vi "MNIST_weight print_OLED_sub.vi"(1 "최소값":dbl=-255.0, 2 "최대값":dbl=255.0, 3 "배열":dbl[][](array[numeric])=[[139.0, 142.0, 145.0, 142.0, 138.0, 139.0, 139.0, 139.0, 139.0, 142.0, 144.0, 141.0, 136.0, 140.0, 145.0, 145.0, 145.0, 145.0, 145.0, 144.0, 141.0, 139.0, 142.0, 144.0, 146.0, 147.0, 142.0, 143.0], [140.0, 138.0, 145.0, 143.0, 144.0, 146.0, 141.0, 136.0, 133.0, 128.0, 125.0, 113.0, 121.0, 115.0, 124.0, 119.0, 122.0, 120.0, 128.0, 126.0, 119.0, 119.0, 122.0, 119.0, 142.0, 138.0, 146.0, 141.0], [142.0, 138.0, 138.0, 124.0, 126.0, 139.0, 135.0, 126.0, 125.0, 125.0, 108.0, 106.0, 104.0, 105.0, 107.0, 105.0, 105.0, 95.0, 111.0, 108.0, 114.0, 117.0, 117.0, 114.0, 144.0, 145.0, 139.0, 141.0], [141.0, 139.0, 144.0, 120.0, 125.0, 121.0, 123.0, 114.0, 118.0, 113.0, 91.0, 75.0, 54.0, 54.0, 35.0, 37.0, 51.0, 92.0, 132.0, 131.0, 108.0, 104.0, 127.0, 131.0, 133.0, 141.0, 143.0, 142.0], [138.0, 138.0, 143.0, 128.0, 142.0, 119.0, 109.0, 82.0, 79.0, 51.0, 46.0, 87.0, 87.0, 91.0, 98.0, 84.0, 77.0, 80.0, 88.0, 11.0, 9.0, 24.0, 68.0, 80.0, 105.0, 134.0, 135.0, 138.0], [138.0, 143.0, 144.0, 124.0, 121.0, 92.0, 54.0, 107.0, 125.0, 115.0, 127.0, 153.0, 148.0, 149.0, 131.0, 138.0, 113.0, 121.0, 123.0, 128.0, 130.0, 117.0, 104.0, 12.0, 36.0, 95.0, 118.0, 136.0], [147.0, 130.0, 114.0, 116.0, 93.0, 73.0, 115.0, 125.0, 129.0, 145.0, 145.0, 155.0, 156.0, 162.0, 162.0, 154.0, 161.0, 165.0, 163.0, 147.0, 149.0, 139.0, 124.0, 100.0, 95.0, 120.0, 99.0, 121.0], [143.0, 115.0, 108.0, 95.0, 81.0, 95.0, 125.0, 120.0, 141.0, 146.0, 145.0, 150.0, 159.0, 170.0, 166.0, 174.0, 170.0, 155.0, 150.0, 151.0, 147.0, 146.0, 137.0, 130.0, 100.0, 96.0, 88.0, 113.0], [129.0, 96.0, 89.0, 92.0, 110.0, 127.0, 137.0, 125.0, 148.0, 137.0, 140.0, 134.0, 133.0, 151.0, 160.0, 157.0, 148.0, 148.0, 145.0, 143.0, 137.0, 151.0, 133.0, 118.0, 113.0, 97.0, 88.0, 127.0], [122.0, 109.0, 83.0, 116.0, 119.0, 139.0, 151.0, 144.0, 146.0, 141.0, 150.0, 142.0, 145.0, 146.0, 152.0, 156.0, 142.0, 143.0, 146.0, 140.0, 141.0, 129.0, 133.0, 117.0, 119.0, 96.0, 88.0, 114.0], [126.0, 110.0, 84.0, 120.0, 126.0, 145.0, 152.0, 145.0, 147.0, 145.0, 146.0, 148.0, 149.0, 134.0, 137.0, 134.0, 141.0, 144.0, 146.0, 139.0, 142.0, 138.0, 135.0, 124.0, 101.0, 121.0, 90.0, 116.0], [123.0, 107.0, 95.0, 117.0, 133.0, 153.0, 150.0, 148.0, 162.0, 153.0, 157.0, 162.0, 142.0, 136.0, 142.0, 153.0, 157.0, 159.0, 158.0, 153.0, 163.0, 157.0, 149.0, 127.0, 106.0, 106.0, 107.0, 125.0], [129.0, 97.0, 102.0, 122.0, 159.0, 155.0, 158.0, 154.0, 153.0, 157.0, 158.0, 151.0, 127.0, 144.0, 149.0, 159.0, 159.0, 167.0, 159.0, 161.0, 160.0, 158.0, 152.0, 164.0, 85.0, 43.0, 92.0, 124.0], [132.0, 112.0, 103.0, 130.0, 176.0, 158.0, 154.0, 155.0, 155.0, 149.0, 152.0, 139.0, 127.0, 146.0, 156.0, 158.0, 169.0, 160.0, 161.0, 163.0, 158.0, 161.0, 150.0, 125.0, 53.0, 76.0, 111.0, 138.0], [124.0, 122.0, 97.0, 148.0, 159.0, 139.0, 152.0, 150.0, 143.0, 145.0, 145.0, 139.0, 135.0, 148.0, 145.0, 160.0, 163.0, 161.0, 152.0, 152.0, 158.0, 151.0, 142.0, 102.0, 32.0, 101.0, 124.0, 140.0], [125.0, 146.0, 91.0, 140.0, 142.0, 145.0, 143.0, 142.0, 150.0, 137.0, 147.0, 149.0, 138.0, 136.0, 137.0, 151.0, 158.0, 156.0, 149.0, 148.0, 146.0, 142.0, 141.0, 107.0, 48.0, 96.0, 136.0, 125.0], [126.0, 132.0, 109.0, 132.0, 142.0, 144.0, 134.0, 145.0, 147.0, 132.0, 148.0, 149.0, 139.0, 135.0, 137.0, 148.0, 159.0, 159.0, 151.0, 134.0, 134.0, 126.0, 140.0, 115.0, 48.0, 72.0, 115.0, 113.0], [140.0, 124.0, 113.0, 124.0, 112.0, 122.0, 131.0, 145.0, 145.0, 143.0, 147.0, 143.0, 143.0, 137.0, 142.0, 154.0, 146.0, 146.0, 142.0, 140.0, 134.0, 131.0, 126.0, 109.0, 58.0, 105.0, 119.0, 115.0], [150.0, 127.0, 113.0, 108.0, 95.0, 110.0, 135.0, 140.0, 138.0, 133.0, 156.0, 149.0, 126.0, 128.0, 152.0, 150.0, 138.0, 143.0, 133.0, 135.0, 140.0, 125.0, 127.0, 99.0, 54.0, 104.0, 104.0, 123.0], [144.0, 119.0, 81.0, 113.0, 105.0, 115.0, 132.0, 143.0, 132.0, 117.0, 130.0, 123.0, 128.0, 134.0, 132.0, 132.0, 135.0, 133.0, 129.0, 139.0, 139.0, 126.0, 121.0, 113.0, 93.0, 121.0, 121.0, 127.0], [138.0, 124.0, 108.0, 119.0, 122.0, 129.0, 121.0, 116.0, 129.0, 110.0, 101.0, 108.0, 114.0, 129.0, 128.0, 126.0, 134.0, 134.0, 125.0, 134.0, 127.0, 113.0, 126.0, 125.0, 149.0, 163.0, 115.0, 142.0], [142.0, 124.0, 106.0, 97.0, 137.0, 138.0, 126.0, 127.0, 133.0, 137.0, 133.0, 124.0, 124.0, 127.0, 131.0, 132.0, 132.0, 126.0, 125.0, 125.0, 131.0, 135.0, 124.0, 126.0, 154.0, 141.0, 116.0, 141.0], [141.0, 138.0, 91.0, 127.0, 143.0, 126.0, 127.0, 127.0, 147.0, 146.0, 150.0, 146.0, 146.0, 138.0, 144.0, 129.0, 137.0, 128.0, 125.0, 118.0, 136.0, 134.0, 143.0, 151.0, 149.0, 141.0, 105.0, 143.0], [144.0, 146.0, 107.0, 132.0, 112.0, 128.0, 123.0, 133.0, 145.0, 135.0, 144.0, 139.0, 140.0, 138.0, 142.0, 137.0, 133.0, 138.0, 133.0, 139.0, 144.0, 146.0, 164.0, 161.0, 152.0, 122.0, 115.0, 138.0], [147.0, 142.0, 120.0, 97.0, 138.0, 153.0, 143.0, 152.0, 143.0, 127.0, 140.0, 130.0, 134.0, 124.0, 127.0, 139.0, 138.0, 146.0, 141.0, 140.0, 154.0, 148.0, 162.0, 172.0, 129.0, 113.0, 122.0, 142.0], [144.0, 146.0, 161.0, 97.0, 143.0, 175.0, 160.0, 153.0, 161.0, 148.0, 151.0, 143.0, 144.0, 150.0, 152.0, 145.0, 152.0, 150.0, 160.0, 156.0, 180.0, 174.0, 142.0, 146.0, 127.0, 124.0, 124.0, 141.0], [140.0, 146.0, 142.0, 158.0, 183.0, 178.0, 184.0, 180.0, 175.0, 178.0, 169.0, 168.0, 176.0, 172.0, 183.0, 161.0, 165.0, 168.0, 174.0, 159.0, 170.0, 154.0, 145.0, 151.0, 152.0, 132.0, 147.0, 138.0], [141.0, 145.0, 138.0, 145.0, 116.0, 115.0, 145.0, 150.0, 153.0, 150.0, 143.0, 142.0, 144.0, 96.0, 150.0, 141.0, 132.0, 110.0, 139.0, 123.0, 146.0, 133.0, 123.0, 118.0, 147.0, 138.0, 147.0, 140.0], [138.0, 0.0, 0.0, 0.0, 0.0, 0.0, 0.0, 0.0, 0.0, 0.0, 0.0, 0.0, 0.0, 0.0, 0.0, 0.0, 0.0, 0.0, 0.0, 0.0, 0.0, 0.0, 0.0, 0.0, 0.0, 0.0, 0.0, 0.0]]) -> (0 "MNIST_Input":dbl[][](graph)=[[139.0, 142.0, 145.0, 142.0, 138.0, 139.0, 139.0, 139.0, 139.0, 142.0, 144.0, 141.0, 136.0, 140.0, 145.0, 145.0, 145.0, 145.0, 145.0, 144.0, 141.0, 139.0, 142.0, 144.0, 146.0, 147.0, 142.0, 143.0], [140.0, 138.0, 145.0, 143.0, 144.0, 146.0, 141.0, 136.0, 133.0, 128.0, 125.0, 113.0, 121.0, 115.0, 124.0, 119.0, 122.0, 120.0, 128.0, 126.0, 119.0, 119.0, 122.0, 119.0, 142.0, 138.0, 146.0, 141.0], [142.0, 138.0, 138.0, 124.0, 126.0, 139.0, 135.0, 126.0, 125.0, 125.0, 108.0, 106.0, 104.0, 105.0, 107.0, 105.0, 105.0, 95.0, 111.0, 108.0, 114.0, 117.0, 117.0, 114.0, 144.0, 145.0, 139.0, 141.0], [141.0, 139.0, 144.0, 120.0, 125.0, 121.0, 123.0, 114.0, 118.0, 113.0, 91.0, 75.0, 54.0, 54.0, 35.0, 37.0, 51.0, 92.0, 132.0, 131.0, 108.0, 104.0, 127.0, 131.0, 133.0, 141.0, 143.0, 142.0], [138.0, 138.0, 143.0, 128.0, 142.0, 119.0, 109.0, 82.0, 79.0, 51.0, 46.0, 87.0, 87.0, 91.0, 98.0, 84.0, 77.0, 80.0, 88.0, 11.0, 9.0, 24.0, 68.0, 80.0, 105.0, 134.0, 135.0, 138.0], [138.0, 143.0, 144.0, 124.0, 121.0, 92.0, 54.0, 107.0, 125.0, 115.0, 127.0, 153.0, 148.0, 149.0, 131.0, 138.0, 113.0, 121.0, 123.0, 128.0, 130.0, 117.0, 104.0, 12.0, 36.0, 95.0, 118.0, 136.0], [147.0, 130.0, 114.0, 116.0, 93.0, 73.0, 115.0, 125.0, 129.0, 145.0, 145.0, 155.0, 156.0, 162.0, 162.0, 154.0, 161.0, 165.0, 163.0, 147.0, 149.0, 139.0, 124.0, 100.0, 95.0, 120.0, 99.0, 121.0], [143.0, 115.0, 108.0, 95.0, 81.0, 95.0, 125.0, 120.0, 141.0, 146.0, 145.0, 150.0, 159.0, 170.0, 166.0, 174.0, 170.0, 155.0, 150.0, 151.0, 147.0, 146.0, 137.0, 130.0, 100.0, 96.0, 88.0, 113.0], [129.0, 96.0, 89.0, 92.0, 110.0, 127.0, 137.0, 125.0, 148.0, 137.0, 140.0, 134.0, 133.0, 151.0, 160.0, 157.0, 148.0, 148.0, 145.0, 143.0, 137.0, 151.0, 133.0, 118.0, 113.0, 97.0, 88.0, 127.0], [122.0, 109.0, 83.0, 116.0, 119.0, 139.0, 151.0, 144.0, 146.0, 141.0, 150.0, 142.0, 145.0, 146.0, 152.0, 156.0, 142.0, 143.0, 146.0, 140.0, 141.0, 129.0, 133.0, 117.0, 119.0, 96.0, 88.0, 114.0], [126.0, 110.0, 84.0, 120.0, 126.0, 145.0, 152.0, 145.0, 147.0, 145.0, 146.0, 148.0, 149.0, 134.0, 137.0, 134.0, 141.0, 144.0, 146.0, 139.0, 142.0, 138.0, 135.0, 124.0, 101.0, 121.0, 90.0, 116.0], [123.0, 107.0, 95.0, 117.0, 133.0, 153.0, 150.0, 148.0, 162.0, 153.0, 157.0, 162.0, 142.0, 136.0, 142.0, 153.0, 157.0, 159.0, 158.0, 153.0, 163.0, 157.0, 149.0, 127.0, 106.0, 106.0, 107.0, 125.0], [129.0, 97.0, 102.0, 122.0, 159.0, 155.0, 158.0, 154.0, 153.0, 157.0, 158.0, 151.0, 127.0, 144.0, 149.0, 159.0, 159.0, 167.0, 159.0, 161.0, 160.0, 158.0, 152.0, 164.0, 85.0, 43.0, 92.0, 124.0], [132.0, 112.0, 103.0, 130.0, 176.0, 158.0, 154.0, 155.0, 155.0, 149.0, 152.0, 139.0, 127.0, 146.0, 156.0, 158.0, 169.0, 160.0, 161.0, 163.0, 158.0, 161.0, 150.0, 125.0, 53.0, 76.0, 111.0, 138.0], [124.0, 122.0, 97.0, 148.0, 159.0, 139.0, 152.0, 150.0, 143.0, 145.0, 145.0, 139.0, 135.0, 148.0, 145.0, 160.0, 163.0, 161.0, 152.0, 152.0, 158.0, 151.0, 142.0, 102.0, 32.0, 101.0, 124.0, 140.0], [125.0, 146.0, 91.0, 140.0, 142.0, 145.0, 143.0, 142.0, 150.0, 137.0, 147.0, 149.0, 138.0, 136.0, 137.0, 151.0, 158.0, 156.0, 149.0, 148.0, 146.0, 142.0, 141.0, 107.0, 48.0, 96.0, 136.0, 125.0], [126.0, 132.0, 109.0, 132.0, 142.0, 144.0, 134.0, 145.0, 147.0, 132.0, 148.0, 149.0, 139.0, 135.0, 137.0, 148.0, 159.0, 159.0, 151.0, 134.0, 134.0, 126.0, 140.0, 115.0, 48.0, 72.0, 115.0, 113.0], [140.0, 124.0, 113.0, 124.0, 112.0, 122.0, 131.0, 145.0, 145.0, 143.0, 147.0, 143.0, 143.0, 137.0, 142.0, 154.0, 146.0, 146.0, 142.0, 140.0, 134.0, 131.0, 126.0, 109.0, 58.0, 105.0, 119.0, 115.0], [150.0, 127.0, 113.0, 108.0, 95.0, 110.0, 135.0, 140.0, 138.0, 133.0, 156.0, 149.0, 126.0, 128.0, 152.0, 150.0, 138.0, 143.0, 133.0, 135.0, 140.0, 125.0, 127.0, 99.0, 54.0, 104.0, 104.0, 123.0], [144.0, 119.0, 81.0, 113.0, 105.0, 115.0, 132.0, 143.0, 132.0, 117.0, 130.0, 123.0, 128.0, 134.0, 132.0, 132.0, 135.0, 133.0, 129.0, 139.0, 139.0, 126.0, 121.0, 113.0, 93.0, 121.0, 121.0, 127.0], [138.0, 124.0, 108.0, 119.0, 122.0, 129.0, 121.0, 116.0, 129.0, 110.0, 101.0, 108.0, 114.0, 129.0, 128.0, 126.0, 134.0, 134.0, 125.0, 134.0, 127.0, 113.0, 126.0, 125.0, 149.0, 163.0, 115.0, 142.0], [142.0, 124.0, 106.0, 97.0, 137.0, 138.0, 126.0, 127.0, 133.0, 137.0, 133.0, 124.0, 124.0, 127.0, 131.0, 132.0, 132.0, 126.0, 125.0, 125.0, 131.0, 135.0, 124.0, 126.0, 154.0, 141.0, 116.0, 141.0], [141.0, 138.0, 91.0, 127.0, 143.0, 126.0, 127.0, 127.0, 147.0, 146.0, 150.0, 146.0, 146.0, 138.0, 144.0, 129.0, 137.0, 128.0, 125.0, 118.0, 136.0, 134.0, 143.0, 151.0, 149.0, 141.0, 105.0, 143.0], [144.0, 146.0, 107.0, 132.0, 112.0, 128.0, 123.0, 133.0, 145.0, 135.0, 144.0, 139.0, 140.0, 138.0, 142.0, 137.0, 133.0, 138.0, 133.0, 139.0, 144.0, 146.0, 164.0, 161.0, 152.0, 122.0, 115.0, 138.0], [147.0, 142.0, 120.0, 97.0, 138.0, 153.0, 143.0, 152.0, 143.0, 127.0, 140.0, 130.0, 134.0, 124.0, 127.0, 139.0, 138.0, 146.0, 141.0, 140.0, 154.0, 148.0, 162.0, 172.0, 129.0, 113.0, 122.0, 142.0], [144.0, 146.0, 161.0, 97.0, 143.0, 175.0, 160.0, 153.0, 161.0, 148.0, 151.0, 143.0, 144.0, 150.0, 152.0, 145.0, 152.0, 150.0, 160.0, 156.0, 180.0, 174.0, 142.0, 146.0, 127.0, 124.0, 124.0, 141.0], [140.0, 146.0, 142.0, 158.0, 183.0, 178.0, 184.0, 180.0, 175.0, 178.0, 169.0, 168.0, 176.0, 172.0, 183.0, 161.0, 165.0, 168.0, 174.0, 159.0, 170.0, 154.0, 145.0, 151.0, 152.0, 132.0, 147.0, 138.0], [141.0, 145.0, 138.0, 145.0, 116.0, 115.0, 145.0, 150.0, 153.0, 150.0, 143.0, 142.0, 144.0, 96.0, 150.0, 141.0, 132.0, 110.0, 139.0, 123.0, 146.0, 133.0, 123.0, 118.0, 147.0, 138.0, 147.0, 140.0], [138.0, 0.0, 0.0, 0.0, 0.0, 0.0, 0.0, 0.0, 0.0, 0.0, 0.0, 0.0, 0.0, 0.0, 0.0, 0.0, 0.0, 0.0, 0.0, 0.0, 0.0, 0.0, 0.0, 0.0, 0.0, 0.0, 0.0, 0.0]])   [LabVIEW 2021]
panel:
  in  "색선택 3":u32[](array[colorbox])=[16711680, 0, 16711935]
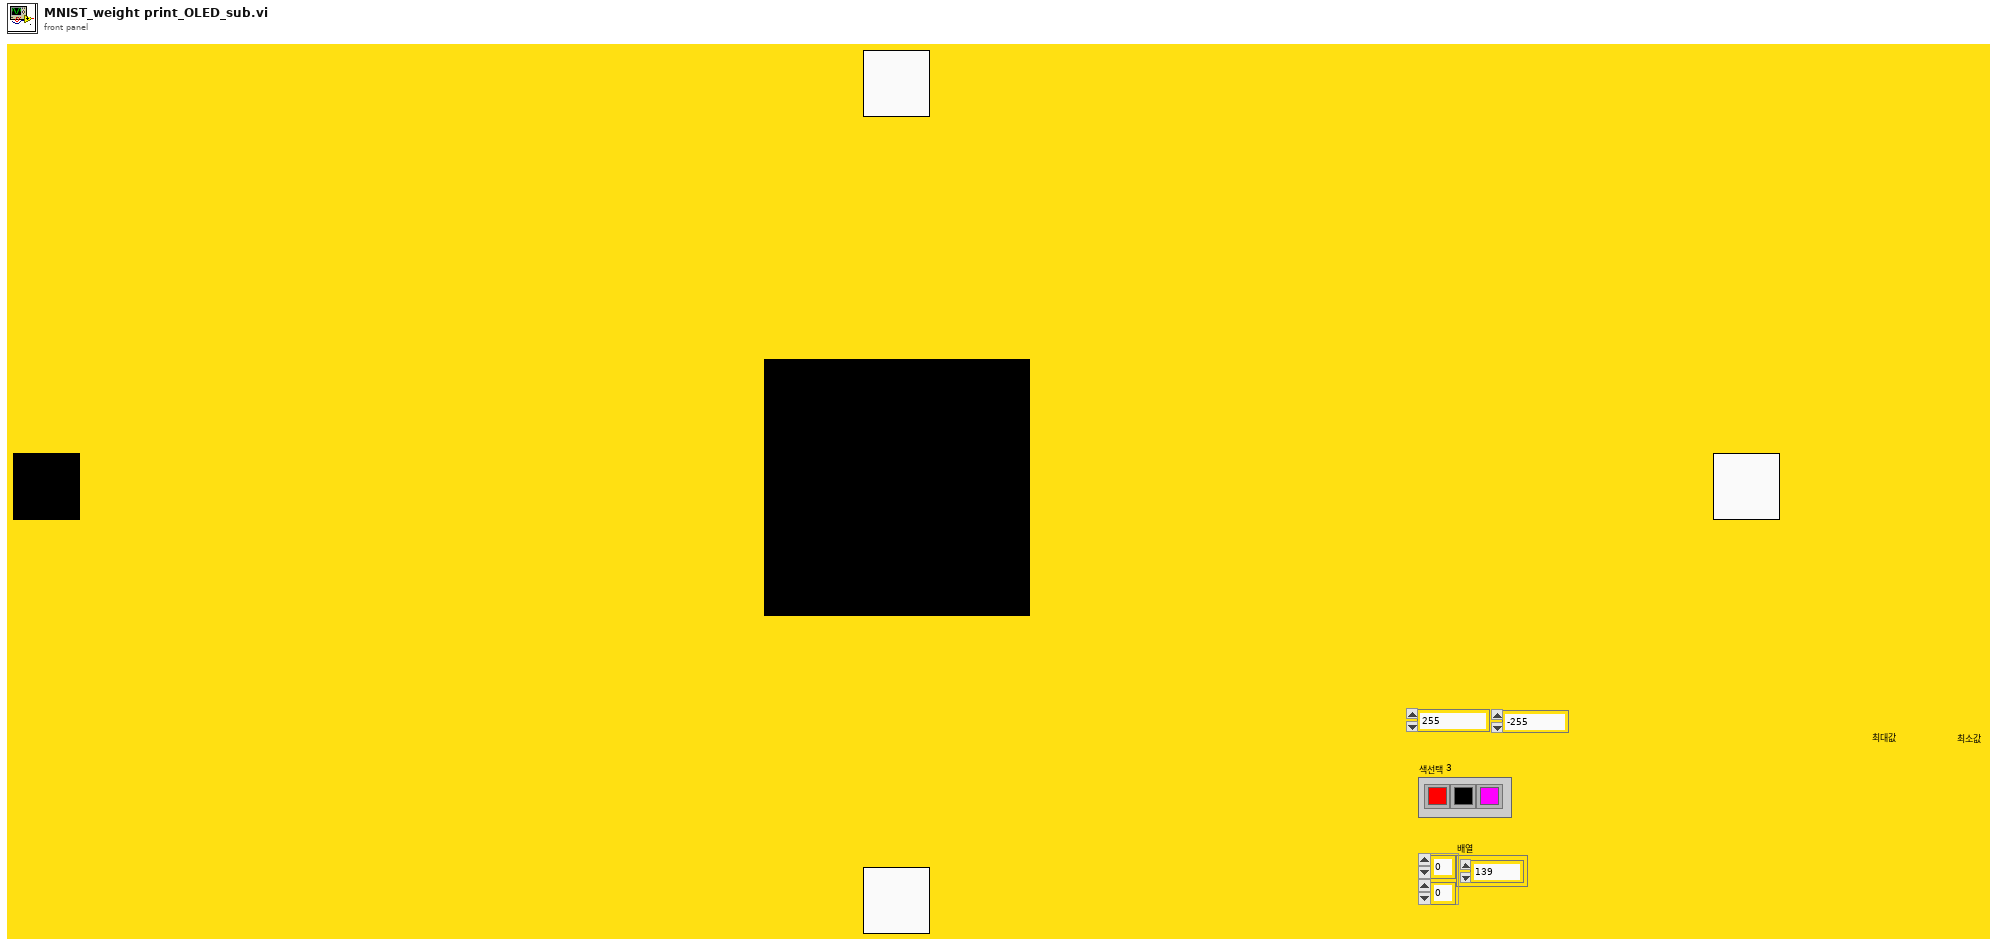
[diagram p1: front panel]
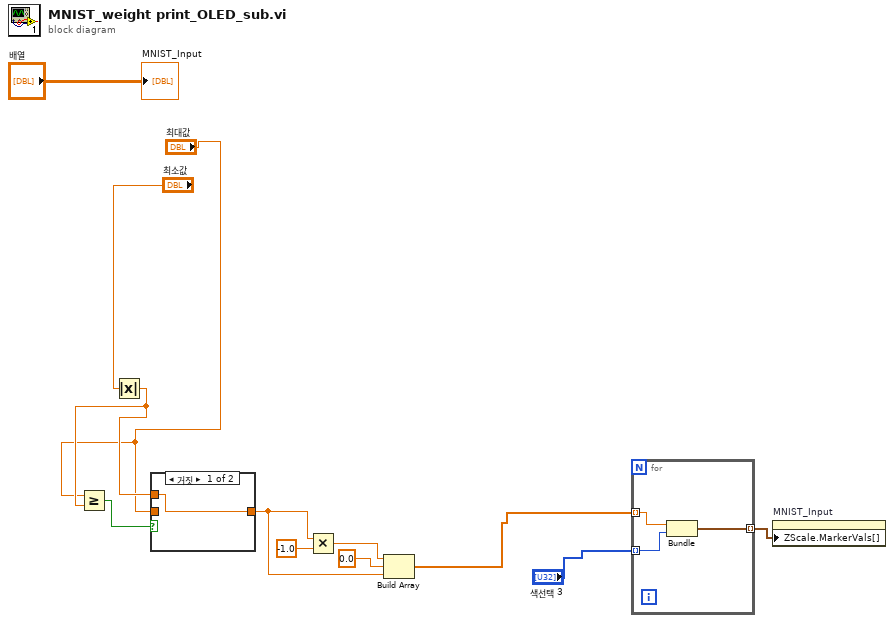
[diagram p0: block diagram]
diagram:
  n1 = Absolute Value(x="최소값") -> (abs(x)=w5:dbl)
  n2 = Greater Or Equal?(x="최대값", y=w5) -> (x >= y?=w11:bool)
  n3 = case shown="거짓" w11 {
    tunnel: "최대값" -> [_ w14]
    tunnel: [w13 w14] -> w7
    tunnel: w5 -> [w13 _]
    frame False {
    }
    frame True {
    }
  }
  n4 = Multiply(x=w7, y=-1.0) -> (x*y=w8:dbl)
  n5 = Build Array(w8, 0.0 ("원소"), w7) -> (w6:dbl[])
  n6 = for {
    tunnel: w6 -> [w17] mode=indexing
    tunnel: "색선택 3" -> [w16] mode=indexing
    tunnel: [w15] -> w3 mode=indexing
    n7 = Bundle("최대값"=w17, "색 상자"=w16) -> (w15:cluster{"최대값":dbl, "색 상자":u32})  [unwired: 1 in]
  }
  n8 = property on="MNIST_Input" class="IntGraph (엄격한)"("ZScale.MarkerVals[]"=w3) -> ()  [unwired: 2 in, 2 out]
  "MNIST_Input" <- "배열"
